vi "ImageAxisToSecondsStatus.vi"(8 "error in (no error)":errorcluster, 11 "Image in":refnum<class "Image.lvclass">) -> (0 "error out":errorcluster, 2 "Intensity x label":string, 3 "Image out":refnum<class "Image.lvclass">)   [LabVIEW 2012, in "Image.lvclass"]
uses:
  classes/Image.lvclass
  classes/Image.lvclass/Image.ctl
  <vilib>/Utility/file.llb/Write To Spreadsheet File (string).vi
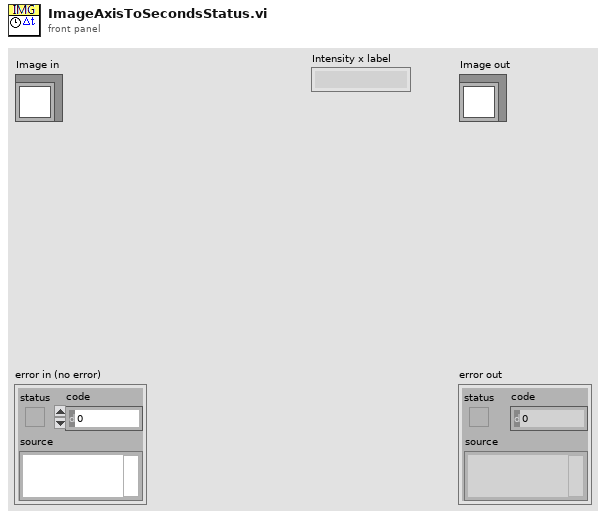
[diagram p1: front panel]
types:
  T1 = typedef "Move Type.ctl" = enum16{"None", "Continuous", "Discrete"}
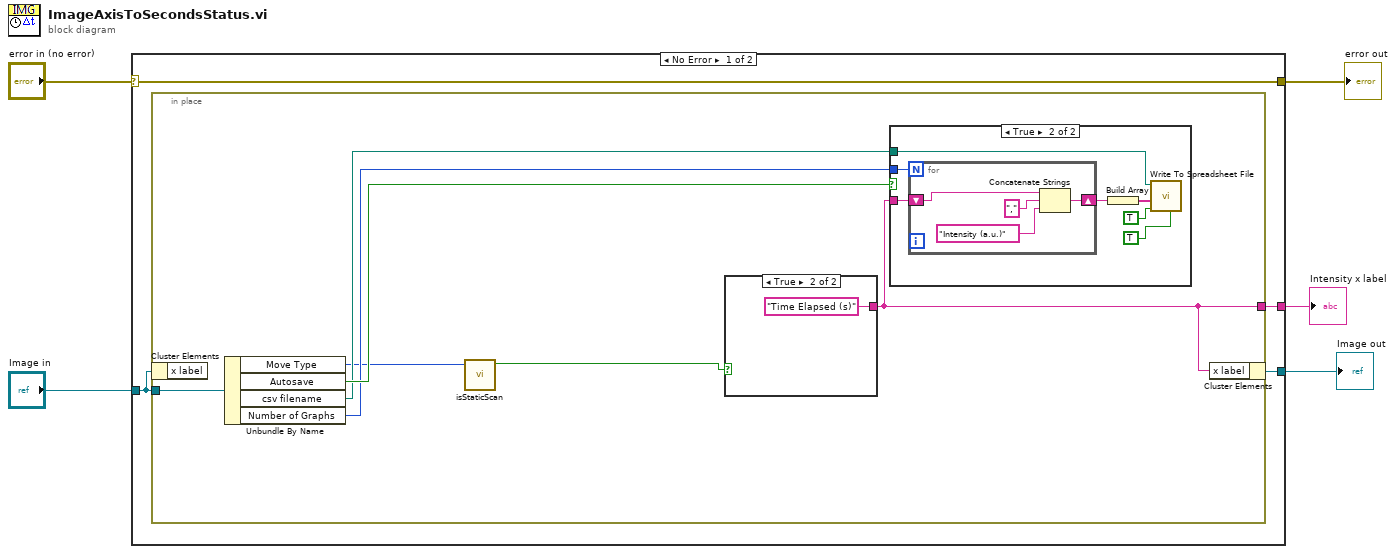
[diagram p0: block diagram]
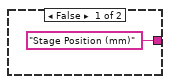
[diagram p3: hidden frame]
diagram:
  n1 = case shown="No Error" "error in (no error)" {
    selector: "error in (no error)" -> [w9 w31]
    tunnel: [w9 w31] -> w4
    tunnel: [w6 w30] -> w2
    tunnel: "Image in" -> [w7 w30]
    tunnel: [w8 _] -> w1
    frame No Error {
      n2 = in-place {
        in-place-border: w7 -> [w16]
        in-place-border: [w12] -> w8
        n3 = in-place-cluster #1(w7) -> ()  [unwired: 1 out]
        n4 = Unbundle By Name(w16) -> ("Move Type"=w10:T1, "Autosave"=w14:bool, "csv filename"=w13:path, "Number of Graphs"=w11:i16)
        n5 = call "isStaticScan.vi"("Move Type"=w10) -> ("Boolean"=w15:bool)  [unwired: 10 in]
        n6 = case shown="True" w15 {
          tunnel: ["Stage Position (mm)" "Time Elapsed (s)"] -> w12
          frame False {
          }
          frame True {
          }
        }
        n7 = case shown="True" w14 {
          tunnel: w13 -> [_ w21]
          tunnel: w12 -> [_ w17]
          tunnel: w11 -> [_ w20]
          frame False {
          }
          frame True {
            n8 = for {
              N: w20 -> [_]
              shift-right: [w24] -> w19
              shift-left: w17 -> [w27]
              n9 = Concatenate Strings(w27, "," ("string"), "Intensity (a.u.)" ("string")) -> (w24:string)
            }
            n10 = Build Array(w19) -> (w18:string[])
            n11 = call-poly <vilib>:"Write To Spreadsheet File.vi"("transpose? (no:F)"=TRUE, "append to file? (new file:F)"=TRUE, "1D data"=w18, "file path (dialog if empty)"=w21) -> ()  [unwired: 4 in, 1 out]
          }
        }
        n12 = in-place-cluster #1("x label"=w12) -> (w6:refnum<class "Image.lvclass">)
      }
    }
    frame Error {
    }
  }
  "error out" <- w4
  "Image out" <- w2
  "Intensity x label" <- w1
